vi "Emballage_BDD_Lecture_BDD_CHIPREG_Test_BDD.vi"(8 "Error in":errorcluster caption="Error in (no error)", 9 "INDICE_PRODUIT_GPAO":i32, 10 "ID_ARTICLE_GPAO":i32, 11 "SN_PRODUIT_AASSIIII":i32) -> (0 "Error out":errorcluster, 3 "Donnee produit":string[](array[string]))   [LabVIEW 2020]
uses:
  Modules/FS/60_FS_Controles/60_FS_SetGet.ctl
  <vilib>/addons/database/Connection.llb/DB Tools Open Connec (Path).vi
  <vilib>/addons/database/Connection.llb/Conn Execute.vi
  <vilib>/addons/database/Recordset.llb/Rec Fetch Recordset Data (R).vi
  <vilib>/addons/database/Recordset.llb/Rec Destroy - Connection.vi
  <vilib>/addons/database/NI_Database_API.lvlib
panel:
  out "données":string[][](array[string])
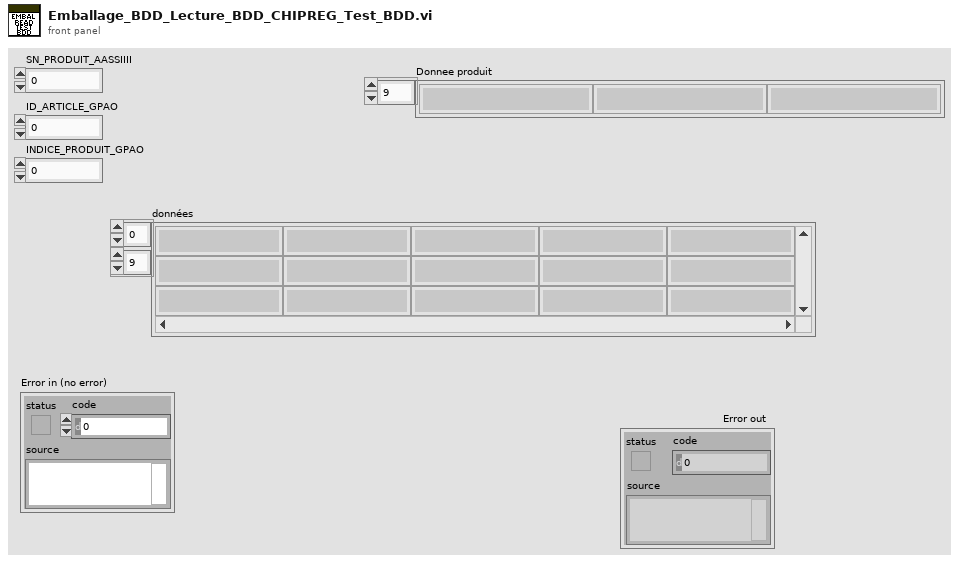
[diagram p1: front panel]
types:
  T1 = typedef "60_FS_SetGet.ctl" = enum16{"set", "get"}
  T2 = typedef "60_FS_CLT_Chemins.ctl" = cluster{"Racine_local":path, "Racine_reseau":path, "Racine_Support_Application":path, "Fichier_Journalisation":path, "Connexion_BDD_VSX":path, "Connexion_BDD_PLZ":path}
  T3 = typedef "NI_Database_API.lvlib/Conn ObjectReference.ctl" = refnum<k1>
  T4 = typedef "NI_Database_API.lvlib/Rec ObjectReference.ctl" = refnum<k1>
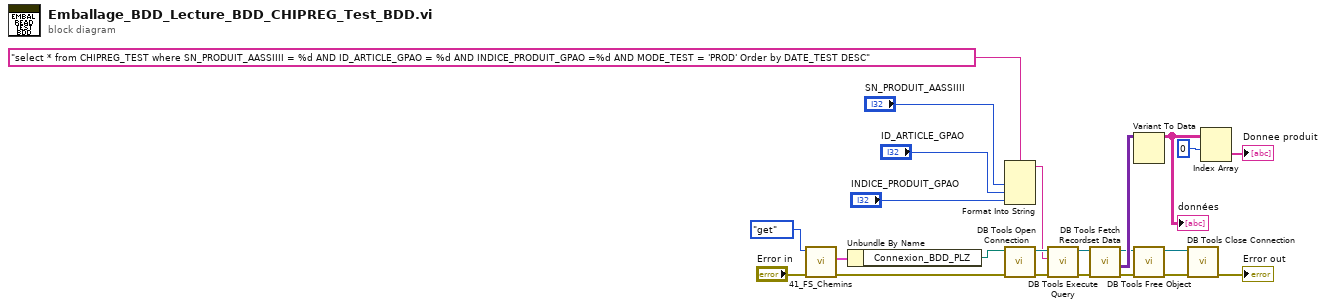
[diagram p0: block diagram]
diagram:
  n1 = call "41_FS_Chemins.vi"("error in (no error)"="Error in", "SetGet"=60_FS_SetGet."get") -> ("error out"=w23:errorcluster, "CLT_Chemins_out"=w21:T2)  [unwired: 8 in]
  n2 = Unbundle By Name(w21) -> ("Connexion_BDD_PLZ"=w3:path)
  n3 = Format Into String(format string="select * from CHIPREG_TEST where SN_PRODUIT_AASSIIII = %d AND ID_ARTICLE_GPAO = %d AND INDICE_PRODUIT_GPAO =%d AND MODE_TEST = 'PROD' Order by DATE_TEST DESC" ("SQL query"), "SN_PRODUIT_AASSIIII", "ID_ARTICLE_GPAO", "INDICE_PRODUIT_GPAO") -> (resulting string=w5:string)  [unwired: 2 in, 1 out]
  n4 = call-poly <vilib>:"DB Tools Open Connection.vi"("error in (no error)"=w23, "connection information"=w3) -> ("error out"=w10:errorcluster, "connection reference"=w9:T3)  [unwired: 6 in]
  n5 = call-poly <vilib>:"DB Tools Execute Query.vi"("error in (no error)"=w10, "SQL query"=w5, "connection reference"=w9) -> ("error out"=w13:errorcluster, "recordset reference"=w15:T4)  [unwired: 5 in]
  n6 = call-poly <vilib>:"DB Tools Fetch Recordset Data.vi"("error in (no error)"=w13, "recordset reference"=w15) -> ("error out"=w14:errorcluster, "recordset data"=w17:variant[][], "recordset reference out"=w16:T4)  [unwired: 3 in]
  n7 = Variant To Data(Variant=w17) -> (data=w18:string[][])  [unwired: 2 in, 1 out]
  "données" <- w18
  n8 = call-poly <vilib>:"DB Tools Free Object.vi"("error in (no error)"=w14, "recordset reference"=w16) -> ("error out"=w11:errorcluster, "connection reference"=w12:T3)  [unwired: 8 in]
  n9 = call <vilib>:"DB Tools Close Connection.vi"("error in (no error)"=w11, "connection reference"=w12) -> ("error out"=→"Error out":errorcluster)  [unwired: 5 in]
  n10 = Index Array(array=w18, index (row)=0 ("indice (ligne)")) -> (element=→"Donnee produit":string[])  [unwired: 1 in]
